vi "Fluigent_MFCS_EZ_Pressure_Modulation.vi"() -> ()   [LabVIEW 2020]
uses:
  <vilib>/DAQmx/read.llb/DAQmx Read (Analog 1D Wfm NChan NSamp).vi
  <userlib>/Fluigent/Fluigent MFCS/FluigentMFCS_Full.llb/MFCS_EZ Detect.vi
  <userlib>/Fluigent/Fluigent MFCS/FluigentMFCS_Full.llb/MFCS_EZ Initialization.vi
  <vilib>/DAQmx/create/channels.llb/DAQmx Create Channel (AI-Voltage-Basic).vi
  <vilib>/DAQmx/configure/timing.llb/DAQmx Timing (Sample Clock).vi
  <vilib>/Waveform/WDTOps.llb/WDT Get XY Value DBL.vi
  <userlib>/Fluigent/Fluigent MFCS/FluigentMFCS_Full.llb/MFCS_EZ Read All Channels Pressure.vi
  <vilib>/DAQmx/miscellaneous.llb/DAQmx Fill In Error Info.vi
  <userlib>/Fluigent/Fluigent MFCS/FluigentMFCS_Full.llb/MFCS_EZ Close.vi
panel:
  out "Measured Waveform 2":dbl(graph)=41.06169018367638
  in  "Sampling Frequency (Hz)":dbl=1000.0
  in  "Voltage Conversion Factor":dbl=100.0 caption="Voltage Conversion Factor (1 V = x mmHg)" format="%0.2f"
  in  "Offset (V)":dbl=0.25 caption="Offset"
  in  "Amplitude (V)":dbl=0.25 caption="Amplitude"
  in  "Phase":dbl
  in  "Reset Signal":bool
  out "Simulated Waveform":waveform(dbl)(graph)={"t0"=timestamp(25.5 s since 1904-01-01), "dt"=0.001, "Y"=[0.25000000000000006, 0.2484292140086103, 0.24685849002916188, 0.24528789007114798, 0.24371747613916567, 0.24214731023046795, 0.2405774543325164, 0.2390079704205338, 0.23743892045505766, 0.23587036637949388, 0.2343023701176717, 0.23273499357139857, 0.23116829861801685, 0.22960234710796062, 0.22803720086231424, 0.22647292167037145, 0.2249095712871963, 0.22334721143118505, 0.2217859037816296, 0.22022570997628257, 0.21866669160892396, 0.2171089102269294, 0.2155524273288405, 0.21399730436193698, 0.21244360271981078, 0.21089138373994232, 0.20934070870127913, 0.20779163882181656, 0.20624423525618102, 0.2046985590932157, 0.20315467135356888, 0.20161263298728496, 0.20007250487139827, 0.19853434780752968, 0.19699822251948637, 0.19546418965086437, 0.19393230976265474, 0.19240264333085239, 0.19087525074406886, 0.18935019230114816, 0.18782752820878634, 0.18630731857915447, 0.1847896234275258, 0.18327450266990614, 0.18176201612066872, 0.1802522234901927, 0.178745184382506, 0.17724095829293204, 0.1757396046057413, 0.17424118259180651, 0.1727457514062632, 0.1712533700861738, 0.16976409754819766, 0.16827799258626439, 0.1667951138692534, 0.16531551993867716, 0.16383926920637076, 0.16236641995218526, 0.16089703032168734, 0.15943115832386356, 0.15796886182883055, 0.15651019856554987, 0.15505522611954975, 0.15360400193065088, 0.15215658329069942, 0.15071302734130484, 0.14927339107158438, 0.14783773131591274, 0.14640610475167903, 0.14497856789704844, 0.1435551771087319, 0.14213598857976026, 0.14072105833726684, 0.1393104422402746, 0.13790419597749198, 0.1365023750651133, 0.1351050348446281, 0.1337122304806354, 0.1323240169586669, 0.13094044908301522, 0.12956158147457125, 0.12818746856866692, 0.12681816461292716, 0.1254537236651273, 0.12409419959105986, 0.1227396460624072, 0.12139011655462345, 0.12004566434482264, 0.11870634250967613, 0.11737220392331649, 0.11604330125525089, 0.11471968696828105, 0.11340141331643278, 0.11208853234289246, 0.11078109587795304, 0.10947915553696735, 0.10818276271831093, 0.10689196860135228, 0.10560682414443315, 0.10432738008285597], "attributes"=variant("NI_ChannelName"=variant(string "Sine"), "NI_ExpIsRelativeTime"=variant(bool TRUE), "NI_ExpStartTimeStamp"=variant(timestamp timestamp(3698011667.1953554 s since 1904-01-01)), "NI_ExpTimeStamp"=variant(timestamp timestamp(3698011692.6953554 s since 1904-01-01)), "NI_ExpXDimension"=variant(string "t"))}
  out "Finished":bool
  out "Time Elapsed (Min)":cluster{dbl, dbl}(slide)={30000.0, 0.43723743000000004} scale=0.0..5.0 scale format="%#_2g"
  out "Dev1 Samples":i32=25838
  out "Running":bool=TRUE
  in  "Signal Frequency (Hz)":dbl=1.0
  in  "Time (min)":dbl(knob)=0.5 min=0.1 max=5.0 step=0.1 scale=0.0..5.0 scale format="%#_2g"
  in  "Session Notes":string[](array[string])=["Sine Wave", "Notes", "test", "1", "1", "junk"]
  out "Analog File Name Fluigent":string="C:\\Users\\kkg5246\\Desktop\\Research\\Fluigent Recordings\\210306_20_33_2506"
  in  "Path for files Fluigent System":path=path "C:/Users/klt8/Documents"
  in  "Stop":bool
  out "Measured Waveform":waveform(dbl)(graph)={"t0"=timestamp(3698011692.933355 s since 1904-01-01), "dt"=0.001, "Y"=[0.23550643619889064, 0.23649361703299174, 0.2351773759206726, 0.23764532800506213, 0.2358354964770165, 0.23846797869870828, 0.23632908689403248, 0.2371517375885986, 0.2369872074497314, 0.23797438828258954, 0.23764532800506213, 0.2368226773108412, 0.23961968966884822, 0.23912609925321165, 0.24175858146755594, 0.2406068704995021, 0.24274576229642394, 0.2409359307762034, 0.24258123215833646, 0.24389747326239697, 0.24307482257253044, 0.2437329431244693, 0.24274576229642394, 0.24521371436499698, 0.24356841298651885, 0.2463654253285757, 0.2437329431244693, 0.24554277464041901, 0.24439106367604302, 0.2462008951909899, 0.24554277464041901, 0.24472012395169299, 0.2463654253285757, 0.24521371436499698, 0.24751713629103952, 0.24587183491575, 0.248339786977832, 0.24685901574119662, 0.248339786977832, 0.2494914979383882, 0.24899790752685735, 0.24965602807551981, 0.249162437664057, 0.25245304040329364, 0.2519594499929849, 0.25557911299719993, 0.25409834176952184, 0.25590817326976967, 0.25607270340602084, 0.25755347463126976, 0.25722441435914944, 0.2562372335422495, 0.25788253490330026, 0.25656629381463936, 0.25870518558298405, 0.25722441435914944, 0.2593633061263275, 0.25788253490330026, 0.26002142666931277, 0.2605150170763167, 0.25919877599052527, 0.25854065544709215, 0.25788253490330026, 0.2601859568050031, 0.2596923663978649, 0.2621603184315435, 0.26002142666931277, 0.2621603184315435, 0.2624893787023209, 0.26446374032511255, 0.2647928005952661, 0.2636410896493393, 0.26446374032511255, 0.26281843897300905, 0.26462827046020043, 0.2624893787023209, 0.26429921019000246, 0.2621603184315435, 0.26380561978453854, 0.26413468005487006, 0.2647928005952661, 0.26577998140519277, 0.2656154512702606, 0.26791887315729135, 0.26577998140519277, 0.26791887315729135, 0.2656154512702606, 0.267096222483851, 0.2664381019446995, 0.26791887315729135, 0.2672607526185834, 0.2661090416749906, 0.2682479334265123, 0.2675898128879817, 0.26972870463691073, 0.26791887315729135, 0.27022229503997874, 0.26808340329191294, 0.2700577649056448, 0.2700577649056448, 0.2698932347712888], "attributes"=variant("NI_ChannelName"=variant(string "Dev1/ai0"), "NI_UnitDescription"=variant(string "Volts"))}
  in  "NI Physical Channels":tag="Dev1/ai0"
  # "Wave type"
  # "Notes"
  # "Simulated Signal Parameters"
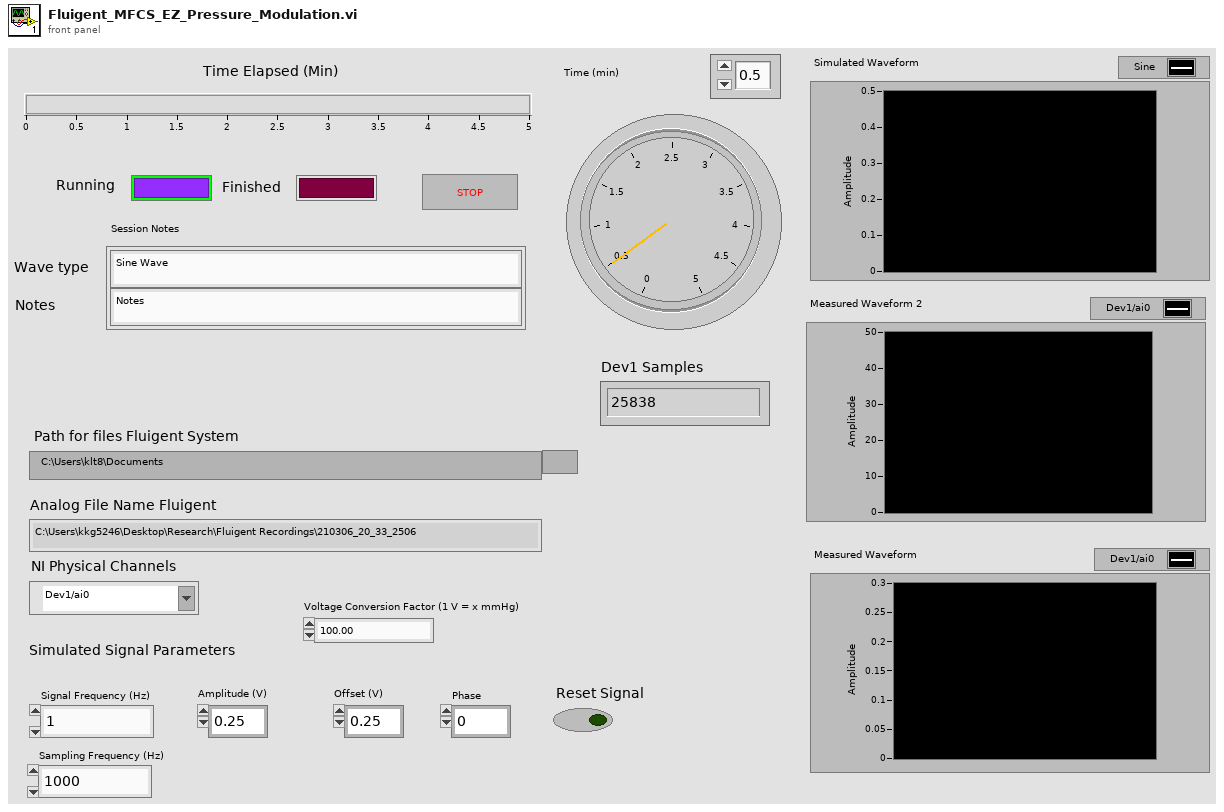
[diagram p1: front panel]
types:
  T1 = enum16{"open", "open or create", "create or replace", "create", "open (read-only)"}
  T2 = typedef "_EZmfcsSN.ctl" = u16
  T3 = typedef "_mfcs_EZ_handle.ctl" = u64
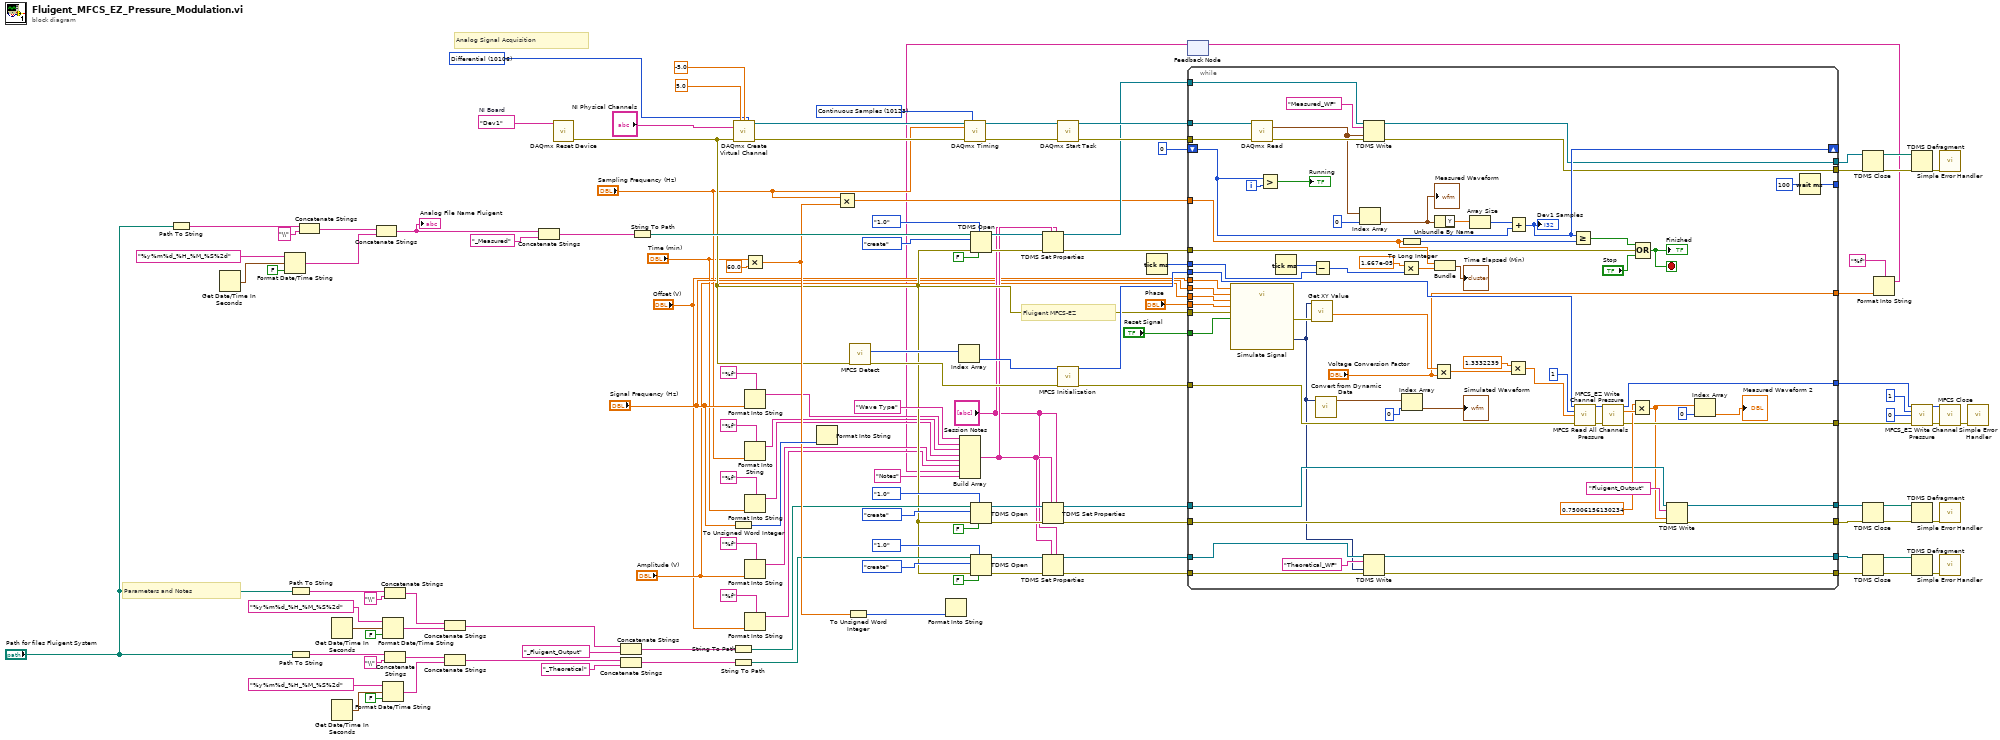
[diagram p0: block diagram]
diagram:
  w87 = tag "Dev1"  # NI Board
  w122 = 10106 items=["default"=-1, "RSE"=10083, "NRSE"=10078, "Differential"=10106, "Pseudodifferential"=12529] ("input terminal configuration")
  w126 = 10123 items=["Finite Samples"=10178, "Continuous Samples"=10123, "Hardware Timed Single Point"=12522] ("sample mode")
  # "Parameters and Notes"
  # "Analog Signal Acquisition"
  # "Fluigent MFCS-EZ"
  n1 = Path To String(path="Path for files Fluigent System") -> (string=w92:string)
  n2 = Get Date/Time In Seconds() -> (seconds since 1Jan1904=w102:timestamp)
  n3 = Format Date/Time String(time format string (%c)="%y%m%d_%H_%M_%S%2d", seconds (now)=w102, UTC format=FALSE) -> (date/time string=w99:string)
  n4 = Path To String(path="Path for files Fluigent System") -> (string=w43:string)
  n5 = Path To String(path="Path for files Fluigent System") -> (string=w59:string)
  n6 = Concatenate Strings(w92, "\\" ("string")) -> (w100:string)
  n7 = Get Date/Time In Seconds() -> (seconds since 1Jan1904=w52:timestamp)
  n8 = Get Date/Time In Seconds() -> (seconds since 1Jan1904=w68:timestamp)
  n9 = Concatenate Strings(w100, w99) -> (w72:string)
  "Analog File Name Fluigent" <- w72
  n10 = Format Date/Time String(time format string (%c)="%y%m%d_%H_%M_%S%2d", seconds (now)=w52, UTC format=FALSE) -> (date/time string=w49:string)
  n11 = Format Date/Time String(time format string (%c)="%y%m%d_%H_%M_%S%2d", seconds (now)=w68, UTC format=FALSE) -> (date/time string=w65:string)
  n12 = Concatenate Strings(w43, "\\" ("string")) -> (w50:string)
  n13 = Concatenate Strings(w59, "\\" ("string")) -> (w66:string)
  n14 = Concatenate Strings(w50, w49) -> (w40:string)
  n15 = Concatenate Strings(w66, w65) -> (w56:string)
  n16 = Concatenate Strings(w72, "_Measured" ("string")) -> (w73:string)
  n17 = call <vilib>:"DAQmx Reset Device.vi"("device in"=w87) -> ("error out"=w37:errorcluster)  [unwired: 14 in]
  n18 = Concatenate Strings(w40, "_Fluigent_Output" ("string")) -> (w41:string)
  n19 = Concatenate Strings(w56, "_Theoretical" ("string")) -> (w57:string)
  n20 = String To Path(string=w73) -> (path=w95:path)
  n21 = To Unsigned Word Integer(number="Signal Frequency (Hz)") -> (unsigned 16bit integer=w78:u16)
  n22 = String To Path(string=w41) -> (path=w45:path)
  n23 = String To Path(string=w57) -> (path=w61:path)
  n24 = call-poly <vilib>:"DAQmx Create Virtual Channel.vi"("maximum value"=5.0, "minimum value"=-5.0, "input terminal configuration"=w122, "physical channels"="NI Physical Channels", "error in"=w37) -> ("task out"=w127:refnum<k21>, "error out"=w125:errorcluster)  [unwired: 4 in, 5 out]
  n25 = Multiply(x="Time (min)", y=60.0) -> (x*y=w77:dbl)
  n26 = Format Into String(format string="%f", "Signal Frequency (Hz)") -> (resulting string=w18:string)  [unwired: 2 in, 1 out]
  n27 = Format Into String(format string="%f", "Sampling Frequency (Hz)") -> (resulting string=w15:string)  [unwired: 2 in, 1 out]
  n28 = Format Into String(format string="%f", "Time (min)") -> (resulting string=w12:string)  [unwired: 2 in, 1 out]
  n29 = Format Into String(format string="%f", "Amplitude (V)") -> (resulting string=w9:string)  [unwired: 2 in, 1 out]
  n30 = Format Into String(format string="%f", "Offset (V)") -> (resulting string=w6:string)  [unwired: 2 in, 1 out]
  n31 = Format Into String(w78) -> ()  [unwired: 3 in, 2 out]
  n32 = Multiply(x="Sampling Frequency (Hz)", y=w77) -> (x*y=w85:dbl)
  n33 = To Unsigned Word Integer(number=w77) -> (unsigned 16bit integer=w76:u16)
  n34 = call-poly <userlib>:"MFCS Detect.vi"("error in (no error)"=w37) -> ("[SN MFCS_EZ]"=w116:T2[], "error out"=w114:errorcluster)  [unwired: 13 in]
  n35 = Format Into String(w76) -> ()  [unwired: 3 in, 2 out]
  n36 = Index Array(array=w116) -> (element=w115:T2)  [unwired: 1 in]
  n37 = call-poly <vilib>:"DAQmx Timing.vi"("task/channels in"=w127, "sample mode"=w126, "rate"="Sampling Frequency (Hz)", "error in"=w125) -> ("task out"=w120:refnum<k21>, "error out"=w119:errorcluster)  [unwired: 3 in, 7 out]
  n38 = TDMS Open(6:FALSE ("disable buffering? (T)"), 7:enum16{"1.0", "2.0"}."1.0" ("file format version (2.0)"), 8:w37, 10:T1."create" ("operation (0:open)"), 11:w95) -> (0:w94:errorcluster, 3:w91:refnum<k34>)  [unwired: 2 in]
  n39 = TDMS Open(6:FALSE ("disable buffering? (T)"), 7:enum16{"1.0", "2.0"}."1.0" ("file format version (2.0)"), 8:w37, 10:T1."create" ("operation (0:open)"), 11:w45) -> (0:w44:errorcluster, 3:w42:refnum<k34>)  [unwired: 2 in]
  n40 = TDMS Open(6:FALSE ("disable buffering? (T)"), 7:enum16{"1.0", "2.0"}."1.0" ("file format version (2.0)"), 8:w37, 10:T1."create" ("operation (0:open)"), 11:w61) -> (0:w60:errorcluster, 3:w58:refnum<k34>)  [unwired: 2 in]
  n41 = call-poly <userlib>:"MFCS Initialization.vi"("SN MFCS_EZ"=w115, "error in (no error)"=w114) -> ("MFCS_EZ_out"=w110:T3, "error out"=w109:errorcluster)  [unwired: 10 in, 2 out]
  n42 = call <vilib>:"DAQmx Start Task.vi"("task/channels in"=w120, "error in"=w119) -> ("task out"=w118:refnum<k21>, "error out"=w117:errorcluster)  [unwired: 12 out]
  n43 = Tick Count (ms)() -> (millisecond timer value=w82:u32)
  n44 = feedback #1() -> (w1:string)  [unwired: 1 in]
  n45 = Build Array("Wave Type", w18, w15, w12, w9, w6, w1, "Notes") -> (w22:string[])
  n46 = TDMS Set Properties(5:"Session Notes", 7:w22, 8:w94, 11:w91) -> (0:w90:errorcluster, 3:w88:refnum<k34>)  [unwired: 4 out]
  n47 = TDMS Set Properties(5:"Session Notes", 7:w22, 8:w44, 11:w42) -> (0:w23:errorcluster, 3:w24:refnum<k34>)  [unwired: 4 out]
  n48 = TDMS Set Properties(5:"Session Notes", 7:w22, 8:w60, 11:w58) -> (0:w29:errorcluster, 3:w36:refnum<k34>)  [unwired: 4 out]
  n49 = while {
    tunnel: w118 -> [w194]
    tunnel: w117 -> [w189]
    tunnel: w110 -> [w190]
    tunnel: w109 -> [w188]
    tunnel: [w159] -> w108
    tunnel: [w187] -> w105
    tunnel: w90 -> [w157]
    tunnel: w88 -> [w158]
    shift-right: [w177] -> _
    shift-left: 0 -> [w178]
    tunnel: w85 -> [w172]
    tunnel: w82 -> [w174]
    tunnel: [w168] -> _
    tunnel: "Signal Frequency (Hz)" -> [w166]
    tunnel: [w162] -> w81
    tunnel: [w161] -> w80
    tunnel: w37 -> [w156]
    tunnel: "Reset Signal" -> [w155]
    tunnel: "Phase" -> [w154]
    tunnel: "Amplitude (V)" -> [w153]
    tunnel: "Offset (V)" -> [w152]
    tunnel: w36 -> [w147]
    tunnel: w29 -> [w146]
    tunnel: [w145] -> w28
    tunnel: [w144] -> w27
    tunnel: [w143] -> w26
    tunnel: [w142] -> w25
    tunnel: w24 -> [w141]
    tunnel: w23 -> [w140]
    tunnel: ["Voltage Conversion Factor"] -> w3
    i -> [w136]
    stop <- w169 stop-if-true
    n50 = call "Simulate Signal"("Offset"=w152, "Reset Signal"=w155, "Frequency"=w166, "Amplitude"=w153, "Phase"=w154, "error in (no error)"=w156) -> ("Sine"=w130:dynamicdata, "error out"=w165:errorcluster)  [unwired: 8 in]
    n51 = call-poly <vilib>:"DAQmx Read.vi"("task/channels in"=w194, "error in"=w189) -> ("data"=w160:waveform(dbl)[], "error out"=w164:errorcluster)  [unwired: 1 in, 11 out]
    n52 = Greater?(x=w178, y=w136) -> (0:→"Running":bool)
    n53 = Tick Count (ms)() -> (millisecond timer value=w175:u32)
    n54 = call-poly <vilib>:"Get XY Value.vi"("error in (no error)"=w165, "waveform in"=w130) -> ("Y value"=w149:dbl)  [unwired: 5 in, 4 out]
    n55 = Subtract(x=w175, y=w174) -> (x-y=w171:u32)
    n56 = call "Convert from Dynamic Data"("Dynamic Data Type"=w130) -> ("Array of Waveform"=w131:waveform(dbl)[])  [unwired: 3 in]
    n57 = Index Array "Index Array"(array=w160, index=0 ("index (row)")) -> (element=w128:waveform(dbl))
    "Measured Waveform" <- w128
    n58 = TDMS Write(0:w158, 5:"Measured_WF", 9:w160, 11:w164) -> (4:w162:refnum<k34>, 15:w161:errorcluster)  [unwired: 2 in, 2 out]
    n59 = TDMS Write(0:w147, 5:"Theoretical_WF", 9:w130, 11:w146) -> (4:w144:refnum<k34>, 15:w145:errorcluster)  [unwired: 2 in, 2 out]
    n60 = Multiply(x=1.667e-05, y=w171) -> (x*y=w176:dbl)
    n61 = To Long Integer(number=w172) -> (32bit integer=w182:i32)
    n62 = Index Array "Index Array"(array=w131, index=0 ("index (row)")) -> (element=→"Simulated Waveform":waveform(dbl))
    n63 = Multiply(x=w149, y="Voltage Conversion Factor") -> (x*y=w151:dbl)
    n64 = Unbundle By Name(w128) -> ("Y"=w180:dbl[])
    n65 = Bundle(w172, w176) -> (→"Time Elapsed (Min)":cluster{dbl, dbl})  [unwired: 1 in]
    n66 = Array Size(array=w180) -> (size(s)=w179:i32)
    n67 = Multiply(x=1.3332239, y=w151) -> (x*y=w148:dbl)
    n68 = Add(x=w179, y=w178) -> (x+y=w177:i32)
    "Dev1 Samples" <- w177
    n69 = Greater Or Equal?(x=w177, y=w182) -> (x >= y?=w181:bool)
    n70 = call <userlib>:"MFCS_EZ Write Channel Pressure.vi"("MFCS_EZ"=w190, "Channel Number (default=1)"=1, "Pressure (mBar)"=w148, "error in (no error)"=w188) -> ("MFCS_EZ out"=w192:T3, "error out"=w193:errorcluster)  [unwired: 10 in]
    n71 = call-poly <userlib>:"MFCS Read All Channels Pressure.vi"("MFCS_EZ"=w192, "error in (no error)"=w193) -> ("MFCS_EZ out"=w187:T3, "All Channels Pressure"=w186:dbl[], "error out"=w159:errorcluster)  [unwired: 11 in]
    n72 = Multiply(x=0.75006156130234, y=w186) -> (x*y=w134:dbl[])
    n73 = Compound Arithmetic op=OR(w181, w157, "Stop") -> (w169:bool)
    "Finished" <- w169
    n74 = TDMS Write(0:w141, 5:"Fluigent_Output", 9:w134, 11:w140) -> (4:w143:refnum<k34>, 15:w142:errorcluster)  [unwired: 2 in, 2 out]
    n75 = Index Array "Index Array"(array=w134, index=0 ("index (row)")) -> (element=→"Measured Waveform 2":dbl)
    n76 = Wait (ms)(milliseconds to wait=u32 100) -> (millisecond timer value=w168:u32)
  }
  n77 = TDMS Close(8:w80, 11:w81) -> (0:w89:errorcluster, 3:w83:path)
  n78 = TDMS Close(8:w25, 11:w26) -> (0:w35:errorcluster, 3:w33:path)
  n79 = TDMS Close(8:w28, 11:w27) -> (0:w32:errorcluster, 3:w30:path)
  n80 = Format Into String(format string="%f", w3) -> (resulting string=w2:string)  [unwired: 2 in, 1 out]
  n81 = feedback-in #1(w2) -> ()
  n82 = TDMS Defragment(4:w89, 7:w83) -> (0:w84:errorcluster)
  n83 = call <userlib>:"MFCS_EZ Write Channel Pressure.vi"("MFCS_EZ"=w105, "Channel Number (default=1)"=1, "Pressure (mBar)"=0, "error in (no error)"=w108) -> ("MFCS_EZ out"=w111:T3, "error out"=w112:errorcluster)  [unwired: 10 in]
  n84 = TDMS Defragment(4:w35, 7:w33) -> (0:w34:errorcluster)
  n85 = TDMS Defragment(4:w32, 7:w30) -> (0:w31:errorcluster)
  n86 = call <vilib>:"Simple Error Handler.vi"("error in (no error)"=w84) -> ()  [unwired: 4 in, 5 out]
  n87 = call-poly <userlib>:"MFCS Close.vi"("MFCS_EZ"=w111, "error in (no error)"=w112) -> ("error out"=w113:errorcluster)  [unwired: 13 in]
  n88 = call <vilib>:"Simple Error Handler.vi"("error in (no error)"=w34) -> ()  [unwired: 4 in, 5 out]
  n89 = call <vilib>:"Simple Error Handler.vi"("error in (no error)"=w31) -> ()  [unwired: 4 in, 5 out]
  n90 = call <vilib>:"Simple Error Handler.vi"("error in (no error)"=w113) -> ()  [unwired: 4 in, 5 out]
